vi "Main.vi"(8 "error in (no error)":errorcluster, 11 "AOTFBase in":refnum<class "AOTF.lvclass">) -> (0 "error out":errorcluster, 3 "component":refnum<class "AOTF.lvclass">)   [LabVIEW 2012, in "AOTF.lvclass"]
doc: "Main VI of the component."
uses:
  AOTF.lvclass
  Controls/laser line enum.ctl
  <vilib>/Distrio/Murmex/Murmex/command_enum.ctl
  AOTF.lvclass/AOTF.ctl
  <vilib>/Distrio/Murmex/InitialiseMessage/InitialiseMessage.lvclass
  <vilib>/Distrio/Murmex/ConfigureMessage/ConfigureMessage.lvclass
  <vilib>/Distrio/Murmex/TerminateMessage/TerminateMessage.lvclass
  <vilib>/Distrio/Murmex/Murmex/update_cluster.ctl
  <vilib>/Distrio/Murmex/GenericMessage/GenericMessage.lvclass
  <vilib>/Distrio/Murmex/Murmex/Set configure at initialise.vi
  <vilib>/Distrio/Murmex/Murmex/Set log reference.vi
  <vilib>/Distrio/Murmex/Murmex/Set VI reference.vi
  <vilib>/Distrio/Murmex/Murmex/Get ID.vi
  <vilib>/Distrio/Murmex/Message/Add or replace parameter.vi
  <vilib>/Distrio/Murmex/Murmex/Murmex.lvclass
  <vilib>/Distrio/Murmex/Message/Message.lvclass
panel:
  in  "button::configure":bool
  in  "button::quit":bool
  out "terminate?":bool=TRUE
  in  "Tab Control":enum32{"Main", "Debug"}(tab)
  in  "PowerPercentage":dbl(knob)=50.0 min=0.0 max=100.0 step=5.0 scale=0.0..100.0
  in  "button::status":bool
  in  "Line On/Off":bool
  in  "button::shutter":bool
  in  "Frequency":T1=103.5 items=["405nm"=150.3, "445nm"=128.71, "491nm"=110.257, "515nm"=103.5, "561nm"=93.2]
  in  "Line number":u32=1 min=1 max=8 step=1
  out "Last read buffer":string="l1F103.500P12.8S1\n\r"
  out "log":string="\r\n11:11:41.970 05/12/2013: initialise from AOTF to AOTF\r\n11:11:42.586 05/12/2013: inform from AOTF to AOTF\r\n11:11:43.913 05/12/2013: update from AOTF to AOTF\r\n11:11:45.142 05/12/2013: generic (shutter_off) from AOTF to AOTF\r\n11:11:45.270 05/12/2013: generic (shutter_on) from AOTF to AOTF\r\n11:11:45.902 05/12/2013: generic (shutter_off) from AOTF to AOTF\r\n11:11:45.932 05/12/2013: inspect from AOTF to AOTF\r\n11:11:48.013 05/12/2013: configure from AOTF to AOTF\r\n11:11:52.003 05/12/2013: inform from AOTF to AOTF\r\n11:11:58.521 05/12/2013: initialise from AOTF to AOTF\r\n11:11:58.561 05/12/2013: inform from AOTF to AOTF\r\n11:11:58.695 05/12/2013: inform from AOTF to AOTF\r\n11:12:02.089 05/12/2013: update from AOTF to AOTF\r\n11:12:02.308 05/12/2013: inspect from AOTF to AOTF\r\n11:12:02.364 05/12/2013: inform from AOTF to AOTF\r\n11:12:05.062 05/12/2013: generic (shutter_on) from AOTF to AOTF\r\n11:12:06.690 05/12/2013: update from AOTF to AOTF\r\n11:12:06.909 05/12/2013: inspect from AOTF to AOTF\r\n11:12:06.964 05/12/2013: inform from AOTF to AOTF\r\n11:12:07.770 05/12/2013: update from AOTF to AOTF\r\n11:12:07.989 05/12/2013: inspect from AOTF to AOTF\r\n11:12:08.044 05/12/2013: inform from AOTF to AOTF\r\n11:12:08.627 05/12/2013: update from AOTF to AOTF\r\n11:12:08.846 05/12/2013: inspect from AOTF to AOTF\r\n11:12:08.900 05/12/2013: inform from AOTF to AOTF\r\n11:12:09.290 05/12/2013: update from AOTF to AOTF\r\n11:12:09.508 05/12/2013: inspect from AOTF to AOTF\r\n11:12:09.563 05/12/2013: inform from AOTF to AOTF\r\n11:12:10.154 05/12/2013: update from AOTF to AOTF\r\n11:12:10.373 05/12/2013: inspect from AOTF to AOTF\r\n11:12:10.430 05/12/2013: inform from AOTF to AOTF\r\n11:12:20.953 05/12/2013: update from AOTF to AOTF\r\n11:12:21.172 05/12/2013: inspect from AOTF to AOTF\r\n11:12:21.227 05/12/2013: inform from AOTF to AOTF\r\n11:12:22.057 05/12/2013: update from AOTF to AOTF\r\n11:12:22.276 05/12/2013: inspect from AOTF to AOTF\r\n11:12:22.330 05/12/2013: inform from AOTF to AOTF\r\n11:12:22.841 05/12/2013: update from AOTF to AOTF\r\n11:12:23.060 05/12/2013: inspect from AOTF to AOTF\r\n11:12:23.114 05/12/2013: inform from AOTF to AOTF\r\n11:12:23.449 05/12/2013: update from AOTF to AOTF\r\n11:12:23.668 05/12/2013: inspect from AOTF to AOTF\r\n11:12:23.724 05/12/2013: inform from AOTF to AOTF\r\n11:12:24.514 05/12/2013: update from AOTF to AOTF\r\n11:12:24.733 05/12/2013: inspect from AOTF to AOTF\r\n11:12:24.789 05/12/2013: inform from AOTF to AOTF\r\n11:12:25.098 05/12/2013: update from AOTF to AOTF\r\n11:12:25.317 05/12/2013: inspect from AOTF to AOTF\r\n11:12:25.371 05/12/2013: inform from AOTF to AOTF\r\n11:12:26.482 05/12/2013: update from AOTF to AOTF\r\n11:12:26.701 05/12/2013: inspect from AOTF to AOTF\r\n11:12:26.755 05/12/2013: inform from AOTF to AOTF\r\n11:12:27.154 05/12/2013: update from AOTF to AOTF\r\n11:12:27.373 05/12/2013: inspect from AOTF to AOTF\r\n11:12:27.428 05/12/2013: inform from AOTF to AOTF\r\n11:12:27.666 05/12/2013: update from AOTF to AOTF\r\n11:12:27.885 05/12/2013: inspect from AOTF to AOTF\r\n11:12:27.944 05/12/2013: inform from AOTF to AOTF\r\n11:12:33.380 05/12/2013: update from AOTF to AOTF\r\n11:12:33.484 05/12/2013: update from AOTF to AOTF\r\n11:12:33.603 05/12/2013: inspect from AOTF to AOTF\r\n11:12:33.611 05/12/2013: update from AOTF to AOTF\r\n11:12:33.684 05/12/2013: update from AOTF to AOTF\r\n11:12:33.740 05/12/2013: update from AOTF to AOTF\r\n11:12:33.827 05/12/2013: inspect from AOTF to AOTF\r\n11:12:33.835 05/12/2013: update from AOTF to AOTF\r\n11:12:33.897 05/12/2013: inform from AOTF to AOTF\r\n11:12:33.903 05/12/2013: update from AOTF to AOTF\r\n11:12:33.940 05/12/2013: update from AOTF to AOTF\r\n11:12:34.085 05/12/2013: update from AOTF to AOTF\r\n11:12:34.119 05/12/2013: inspect from AOTF to AOTF\r\n11:12:34.292 05/12/2013: update from AOTF to AOTF\r\n11:12:34.336 05/12/2013: inspect from AOTF to AOTF\r\n11:12:34.553 05/12/2013: inspect from AOTF to AOTF\r\n11:12:34.608 05/12/2013: inform from AOTF to AOTF\r\n11:12:34.739 05/12/2013: update from AOTF to AOTF\r\n11:12:34.771 05/12/2013: update from AOTF to AOTF\r\n11:12:34.826 05/12/2013: inspect from AOTF to AOTF\r\n11:12:34.834 05/12/2013: update from AOTF to AOTF\r\n11:12:34.867 05/12/2013: update from AOTF to AOTF\r\n11:12:34.931 05/12/2013: update from AOTF to AOTF\r\n11:12:34.979 05/12/2013: update from AOTF to AOTF\r\n11:12:35.003 05/12/2013: update from AOTF to AOTF\r\n11:12:35.027 05/12/2013: update from AOTF to AOTF\r\n11:12:35.041 05/12/2013: update from AOTF to AOTF\r\n11:12:35.051 05/12/2013: inspect from AOTF to AOTF\r\n11:12:35.066 05/12/2013: update from AOTF to AOTF\r\n11:12:35.116 05/12/2013: update from AOTF to AOTF\r\n11:12:35.171 05/12/2013: update from AOTF to AOTF\r\n11:12:35.211 05/12/2013: update from AOTF to AOTF\r\n11:12:35.273 05/12/2013: inspect from AOTF to AOTF\r\n11:12:35.287 05/12/2013: update from AOTF to AOTF\r\n11:12:35.475 05/12/2013: update from AOTF to AOTF\r\n11:12:35.495 05/12/2013: inspect from AOTF to AOTF\r\n11:12:35.549 05/12/2013: inform from AOTF to AOTF\r\n11:12:35.764 05/12/2013: inspect from AOTF to AOTF\r\n11:12:35.819 05/12/2013: inform from AOTF to AOTF\r\n11:12:35.861 05/12/2013: update from AOTF to AOTF\r\n11:12:35.877 05/12/2013: inform from AOTF to AOTF\r\n11:12:35.947 05/12/2013: update from AOTF to AOTF\r\n11:12:36.067 05/12/2013: update from AOTF to AOTF\r\n11:12:36.100 05/12/2013: inspect from AOTF to AOTF\r\n11:12:36.235 05/12/2013: update from AOTF to AOTF\r\n11:12:36.317 05/12/2013: inspect from AOTF to AOTF\r\n11:12:36.371 05/12/2013: inform from AOTF to AOTF\r\n11:12:36.587 05/12/2013: inspect from AOTF to AOTF\r\n11:12:36.771 05/12/2013: update from AOTF to AOTF\r\n11:12:36.804 05/12/2013: inspect from AOTF to AOTF\r\n11:12:37.020 05/12/2013: inspect from AOTF to AOTF\r\n11:12:37.238 05/12/2013: inspect from AOTF to AOTF\r\n11:12:37.456 05/12/2013: inspect from AOTF to AOTF\r\n11:12:37.673 05/12/2013: inspect from AOTF to AOTF\r\n11:12:37.891 05/12/2013: inspect from AOTF to AOTF\r\n11:12:37.946 05/12/2013: inform from AOTF to AOTF\r\n11:12:38.161 05/12/2013: inspect from AOTF to AOTF\r\n11:12:38.379 05/12/2013: inspect from AOTF to AOTF\r\n11:12:38.597 05/12/2013: inspect from AOTF to AOTF\r\n11:12:38.815 05/12/2013: inspect from AOTF to AOTF\r\n11:12:38.871 05/12/2013: inform from AOTF to AOTF\r\n11:12:39.086 05/12/2013: inspect from AOTF to AOTF\r\n11:12:39.303 05/12/2013: inspect from AOTF to AOTF\r\n11:12:39.363 05/12/2013: inform from AOTF to AOTF\r\n11:12:39.417 05/12/2013: inform from AOTF to AOTF\r\n11:12:39.633 05/12/2013: inspect from AOTF to AOTF\r\n11:12:39.852 05/12/2013: inspect from AOTF to AOTF\r\n11:12:40.069 05/12/2013: inspect from AOTF to AOTF\r\n11:12:40.124 05/12/2013: inform from AOTF to AOTF\r\n11:12:40.339 05/12/2013: inspect from AOTF to AOTF\r\n11:12:40.395 05/12/2013: inform from AOTF to AOTF\r\n11:12:40.448 05/12/2013: inform from AOTF to AOTF\r\n11:12:40.663 05/12/2013: inspect from AOTF to AOTF\r\n11:12:40.718 05/12/2013: inform from AOTF to AOTF\r\n11:12:40.770 05/12/2013: inform from AOTF to AOTF\r\n11:12:40.824 05/12/2013: inform from AOTF to AOTF\r\n11:12:40.877 05/12/2013: inform from AOTF to AOTF\r\n11:12:40.930 05/12/2013: inform from AOTF to AOTF\r\n11:12:40.982 05/12/2013: inform from AOTF to AOTF\r\n11:12:41.034 05/12/2013: inform from AOTF to AOTF\r\n11:12:41.092 05/12/2013: inform from AOTF to AOTF\r\n11:12:41.144 05/12/2013: inform from AOTF to AOTF\r\n11:12:41.196 05/12/2013: inform from AOTF to AOTF\r\n11:12:41.249 05/12/2013: inform from AOTF to AOTF\r\n11:12:41.307 05/12/2013: inform from AOTF to AOTF\r\n11:12:41.366 05/12/2013: inform from AOTF to AOTF\r\n11:12:41.424 05/12/2013: inform from AOTF to AOTF\r\n11:12:41.478 05/12/2013: inform from AOTF to AOTF\r\n11:12:41.533 05/12/2013: inform from AOTF to AOTF\r\n11:12:41.589 05/12/2013: inform from AOTF to AOTF\r\n11:12:42.246 05/12/2013: terminate from AOTF to AOTF"
  in  "component ID":string="AOTF"
  in  "button::send":bool
  in  "command":T2
  in  "Generic command":string
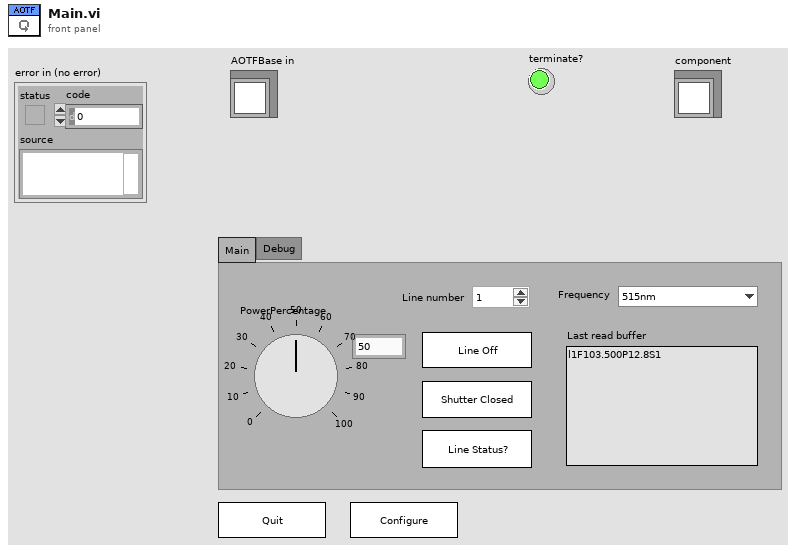
[diagram p1: front panel]
types:
  T1 = typedef "AOTF.lvclass/laser line enum.ctl" = dbl
  T2 = typedef "Murmex.lvlib/Murmex.lvclass/command_enum.ctl" = enum16{"null", "initialise", "reset", "terminate", "acknowledge", "update", "inspect", "inform", "proceed", "start", "stop", "fetch", "configure", "generic"}
  T3 = enum8{"Enabled", "Disabled", "Disabled and Grayed Out"}
  T4 = typedef "Murmex.lvlib/Murmex.lvclass/update_cluster.ctl" = cluster{"target ID":string, "key chains":string[], "values":variant[]}
  T5 = typedef "Murmex.lvclass/command_enum.ctl" = enum16{"null", "initialise", "reset", "terminate", "acknowledge", "update", "inspect", "inform", "proceed", "start", "stop", "fetch", "configure", "generic"}
  T6 = typedef "Murmex.lvclass/Event type enumerations.ctl" = enum16{"before", "after"}
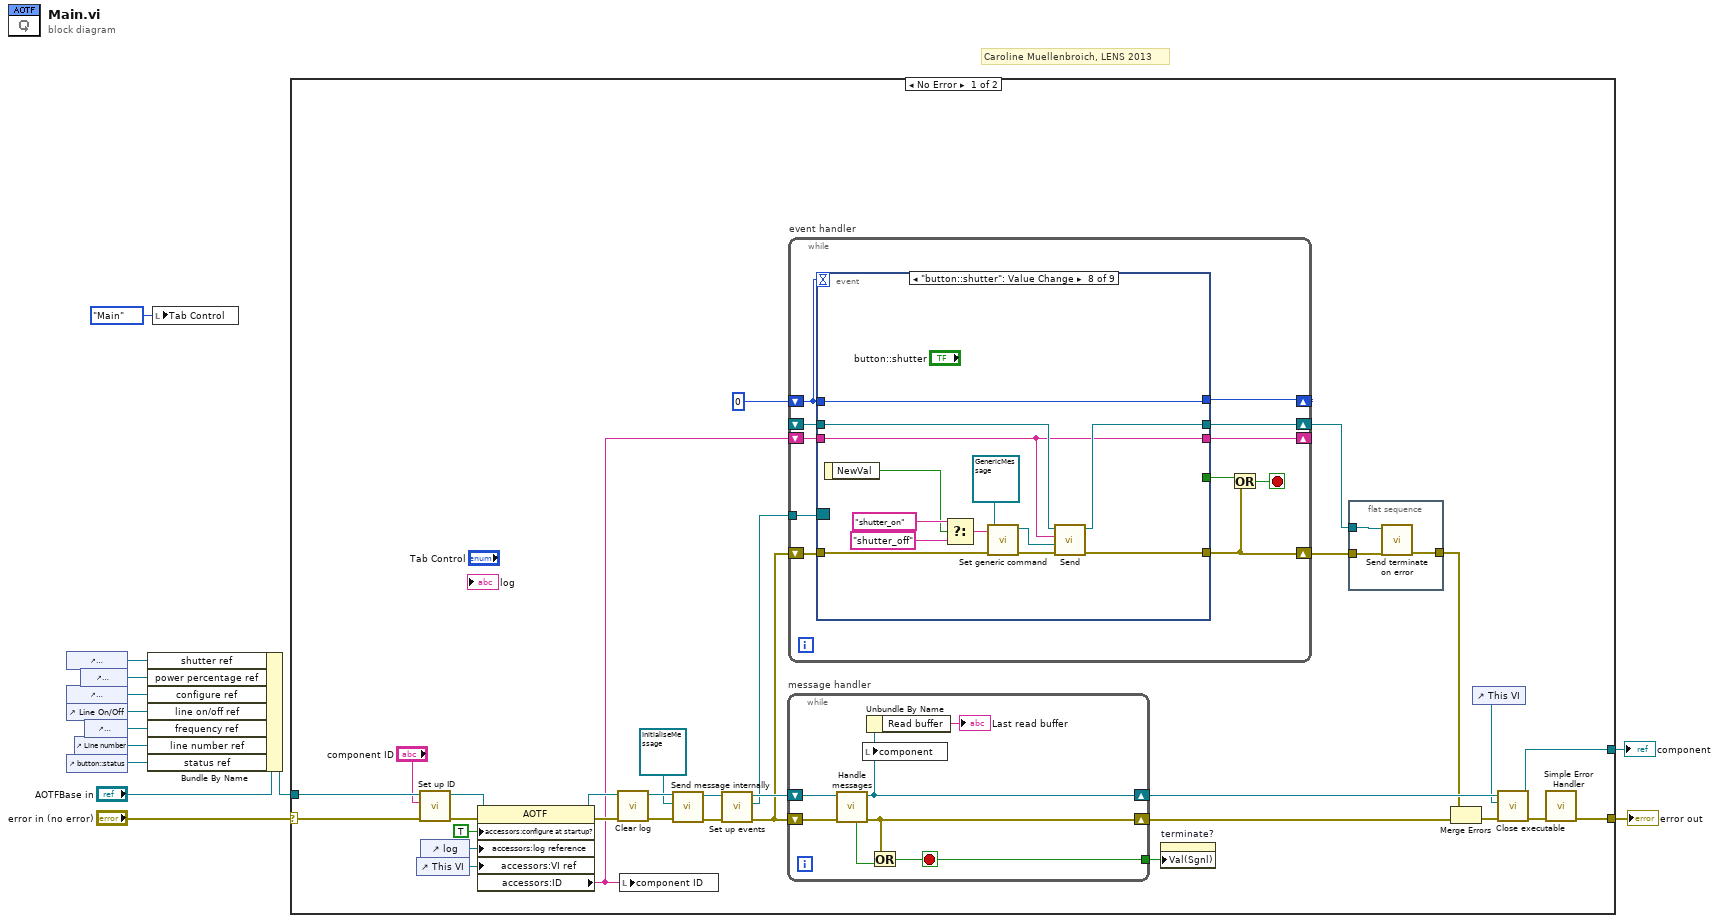
[diagram p0: block diagram]
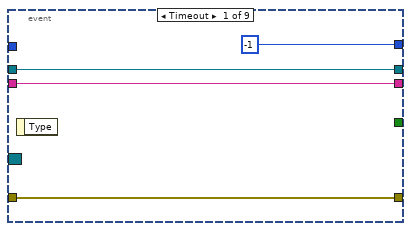
[diagram p2: hidden frame]
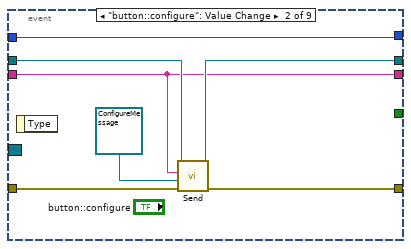
[diagram p3: hidden frame]
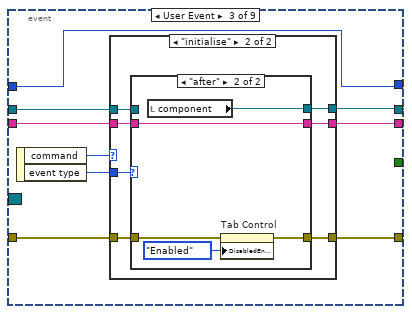
[diagram p4: hidden frame]
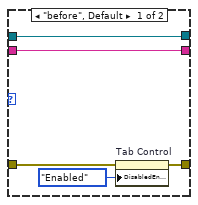
[diagram p6: hidden frame]
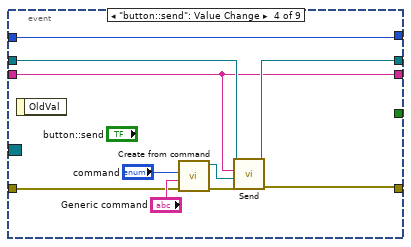
[diagram p7: hidden frame]
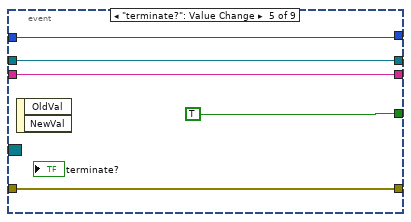
[diagram p8: hidden frame]
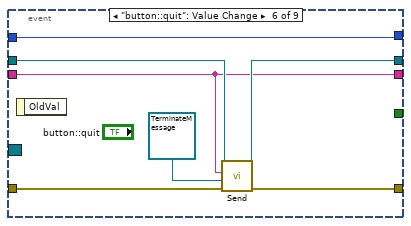
[diagram p9: hidden frame]
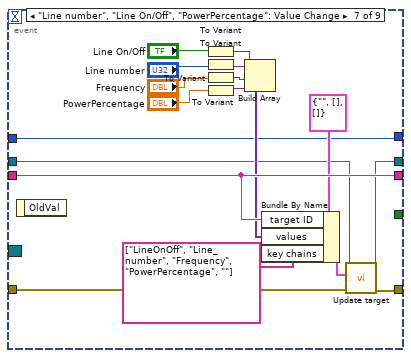
[diagram p10: hidden frame]
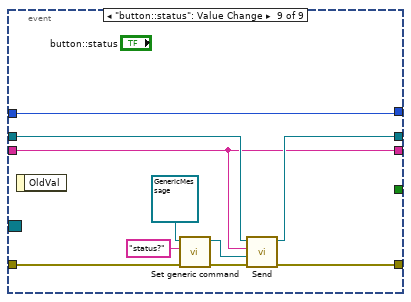
[diagram p11: hidden frame]
diagram:
  # "Caroline Muellenbroich, LENS 2013"
  n1 = control-ref of="button::shutter"() -> (w4:refnum<vi>)
  n2 = control-ref of="button::configure"() -> (w7:refnum<vi>)
  n3 = control-ref of="Line On/Off"() -> (w2:refnum<vi>)
  n4 = control-ref of="button::status"() -> (w1:refnum<vi>)
  n5 = control-ref of="Line number"() -> (w5:refnum<vi>)
  n6 = control-ref of="PowerPercentage"() -> (w3:refnum<vi>)
  n7 = control-ref of="Frequency"() -> (w6:refnum<vi>)
  n8 = Bundle By Name(cluster="AOTFBase in", "shutter ref"=w4, "power percentage ref"=w3, "configure ref"=w7, "line on/off ref"=w2, "frequency ref"=w6, "line number ref"=w5, "status ref"=w1) -> (w8:refnum<class "AOTF.lvclass">)
  n9 = local write "Tab Control"(enum32{"Main", "Debug"}."Main" ("Tab Control")) -> ()
  n10 = case shown="No Error" "error in (no error)" {
    selector: "error in (no error)" -> [w17 w170]
    tunnel: w8 -> [w44 w169]
    tunnel: [w27 w169] -> w13
    tunnel: [w23 w170] -> w12
    frame No Error {
      n11 = control-ref of="This VI"() -> (w39:refnum<vi>)
      n12 = call <vilib>:"Set up ID.vi"("error in (no error)"=w17, "component ID"="component ID", "MurmexBase in"=w44) -> ("error out"=w43:errorcluster, "MurmexBase out"=w42:refnum<class "AOTF.lvclass">)  [unwired: 6 in, 1 out]
      n13 = control-ref of="log"() -> (w40:refnum<vi>)
      n14 = property class="AOTF"(reference=w42, error in=w43, "accessors:configure at startup?"=TRUE ("configure at startup?"), "accessors:log reference"=w40, "accessors:VI ref"=w39) -> (reference out=w36:refnum<class "AOTF.lvclass">, error out=w38:errorcluster, "accessors:ID"=w16:string)
      n15 = call <vilib>:"Clear log.vi"("error in (no error)"=w38, "MurmexBase in"=w36) -> ("error out"=w37:errorcluster, "MurmexBase out"=w35:refnum<class "AOTF.lvclass">)  [unwired: 8 in]
      n16 = local write "component ID"(w16) -> ()
      n17 = call <vilib>:"Send message internally.vi"("error in (no error)"=w37, "Message"=refnum<class "InitialiseMessage.lvclass"> refnum ("Murmex.lvlib:InitialiseMessage"), "Murmex in"=w35) -> ("error out"=w34:errorcluster, "Murmex out"=w33:refnum<class "AOTF.lvclass">)  [unwired: 7 in]
      n18 = call <vilib>:"Set up events.vi"("error in (no error)"=w34, "MurmexBase in"=w33) -> ("error out"=w26:errorcluster, "Event Registration Refnum"=w25:refnum<event-registration>, "MurmexBase out"=w32:refnum<class "AOTF.lvclass">)  [unwired: 7 in]
      n19 = while "message handler" {
        shift-right: [w163] -> w28
        shift-left: w32 -> [w167]
        shift-right: [w166] -> w29
        shift-left: w26 -> [w168]
        tunnel: [w164] -> w24
        stop <- w164 stop-if-true
        n20 = call <vilib>:"Handle messages.vi"("error in (no error)"=w168, "Murmex in"=w167) -> ("error out"=w166:errorcluster, "Murmex out"=w163:refnum<class "AOTF.lvclass">, "terminated?"=w165:bool)  [unwired: 7 in]
        n21 = local write "component"(w163) -> ()
        n22 = Unbundle By Name(w163) -> ("Read buffer"=→"Last read buffer":string)
        n23 = Or(x=w166, y=w165) -> (x .or. y?=w164:bool)
      }
      n24 = while "event handler" {
        tunnel: w25 -> [w58]
        shift-right: [w51] -> w21
        shift-left: w26 -> [w57]
        shift-right: [w53] -> _
        shift-left: w16 -> [w56]
        shift-right: [w55] -> w19
        shift-left: _ -> [w54]
        shift-right: [w49] -> _
        shift-left: 0 -> [w48]
        stop <- w52 stop-if-true
        n25 = event shown="[7] \"button::shutter\": Value Change" {
          selector: w58 -> [_ _ _ _ _ _ _ _ _]
          dyn-events: _ -> [_ _ _ _ _ _ _ _ _]
          timeout: w48 -> [_ _ _ _ _ _ _ _ _]
          tunnel: w57 -> [w60 w69 w76 w105 w113 w120 w137 w149 w159]
          tunnel: [w60 w68 w75 w104 w113 w119 w138 w150 w160] -> w51
          tunnel: w56 -> [w62 w64 w74 w100 w111 w115 w136 w142 w154]
          tunnel: [w61 w66 w73 w102 w110 w117 w130 w146 w156] -> w55
          tunnel: w54 -> [w61 w67 w72 w103 w110 w118 w131 w147 w157]
          tunnel: [w62 w64 w71 w100 w111 w115 w136 w142 w154] -> w53
          tunnel: [_ _ _ _ TRUE _ _ _ _] -> w50
          tunnel: w48 -> [_ w65 w70 w101 w109 w116 w123 w140 w153]
          tunnel: [-1 w65 w70 w101 w109 w116 w123 w140 w153] -> w49
          event Timeout {
            n26 = event-data() -> ()  [unwired: 1 in, 1 out]
          }
          event "button::configure": Value Change {
            n27 = event-data() -> ()  [unwired: 1 in, 1 out]
            n28 = call <vilib>:"Send.vi"("error in (no error)"=w69, "Message"=refnum<class "ConfigureMessage.lvclass"> refnum ("Murmex.lvlib:ConfigureMessage"), "recipient"=w64, "Murmex in"=w67) -> ("error out"=w68:errorcluster, "Murmex out"=w66:refnum<class "Murmex.lvclass">)  [unwired: 6 in]
          }
          event User Event {
            n29 = event-data() -> ("command"=w78:T5, "event type"=w77:T6)  [unwired: 1 in]
            n30 = case shown="\"initialise\"" w78 {
              tunnel: w77 -> [_ w88]
              tunnel: w76 -> [w79 w87]
              tunnel: [w79 w86] -> w75
              tunnel: w74 -> [w81 w85]
              tunnel: [w80 w84] -> w73
              tunnel: w72 -> [w80 w83]
              tunnel: [w81 w82] -> w71
              frame "null", Default {
              }
              frame "initialise" {
                n31 = case shown="\"after\"" w88 {
                  tunnel: [w92 w97] -> w86
                  tunnel: w87 -> [w93 w98]
                  tunnel: w85 -> [w90 w94]
                  tunnel: [w89 w96] -> w84
                  tunnel: w83 -> [w89 _]
                  tunnel: [w90 w94] -> w82
                  frame "before", Default {
                    n32 = property on="Tab Control" class="TabCtl (strict)"(error in=w93, "DisabledEnum"=T3."Enabled" ("Disabled")) -> (error out=w92:errorcluster)  [unwired: 1 in, 1 out]
                  }
                  frame "after" {
                    n33 = local read "component"() -> (w96:refnum<class "AOTF.lvclass">)
                    n34 = property on="Tab Control" class="TabCtl (strict)"(error in=w98, "DisabledEnum"=T3."Enabled" ("Disabled")) -> (error out=w97:errorcluster)  [unwired: 1 in, 1 out]
                  }
                }
              }
            }
          }
          event "button::send": Value Change {
            n35 = event-data() -> ()  [unwired: 1 in, 1 out]
            n36 = call <vilib>:"Create from command.vi"("error in (no error)"=w105, "generic command"="Generic command", "command"="command") -> ("error out"=w107:errorcluster, "Message out"=w106:refnum<class "Message.lvclass">)  [unwired: 7 in]
            n37 = call <vilib>:"Send.vi"("error in (no error)"=w107, "Message"=w106, "recipient"=w100, "Murmex in"=w103) -> ("error out"=w104:errorcluster, "Murmex out"=w102:refnum<class "Murmex.lvclass">)  [unwired: 6 in]
          }
          event "terminate?": Value Change {
            n38 = event-data() -> ()  [unwired: 1 in, 2 out]
          }
          event "button::quit": Value Change {
            n39 = event-data() -> ()  [unwired: 1 in, 1 out]
            n40 = call <vilib>:"Send.vi"("error in (no error)"=w120, "Message"=refnum<class "TerminateMessage.lvclass"> refnum ("Murmex.lvlib:TerminateMessage"), "recipient"=w115, "Murmex in"=w118) -> ("error out"=w119:errorcluster, "Murmex out"=w117:refnum<class "Murmex.lvclass">)  [unwired: 6 in]
          }
          event "Line number", "Line On/Off", "PowerPercentage": Value Change {
            n41 = event-data() -> ()  [unwired: 1 in, 1 out]
            n42 = To Variant(anything="Line On/Off") -> (Variant=w129:variant)
            n43 = To Variant(anything="Line number") -> (Variant=w126:variant)
            n44 = To Variant(anything="Frequency") -> (Variant=w127:variant)
            n45 = To Variant(anything="PowerPercentage") -> (Variant=w128:variant)
            n46 = Build Array(w129, w126, w127, w128) -> (w132:variant[])
            n47 = Bundle By Name(cluster=T4 {"target ID"="", "key chains"=[], "values"=[]} ("update cluster"), "target ID"=w136, "values"=w132, "key chains"=string[] ["LineOnOff", "Line_number", "Frequency", "PowerPercentage", ""]) -> (w135:T4)
            n48 = call <vilib>:"Update target.vi"("error in (no error)"=w137, "update cluster"=w135, "MurmexBase in"=w131) -> ("error out"=w138:errorcluster, "MurmexBase out"=w130:refnum<class "Murmex.lvclass">)  [unwired: 7 in]
          }
          event "button::shutter": Value Change {
            n49 = event-data() -> ("NewVal"=w141:bool)  [unwired: 1 in]
            n50 = Select(t="shutter_on" ("generic command"), s=w141, f="shutter_off" ("generic command")) -> (s? t:f=w143:string)
            n51 = call <vilib>:"Set generic command.vi"("error in (no error)"=w149, "generic command"=w143, "GenericMessage in"=refnum<class "GenericMessage.lvclass"> refnum ("Murmex.lvlib:GenericMessage")) -> ("error out"=w148:errorcluster, "GenericMessage out"=w151:refnum<class "GenericMessage.lvclass">)  [unwired: 7 in]
            n52 = call <vilib>:"Send.vi"("error in (no error)"=w148, "Message"=w151, "recipient"=w142, "Murmex in"=w147) -> ("error out"=w150:errorcluster, "Murmex out"=w146:refnum<class "Murmex.lvclass">)  [unwired: 6 in]
          }
          event "button::status": Value Change {
            n53 = event-data() -> ()  [unwired: 1 in, 1 out]
            n54 = call <vilib>:"Set generic command.vi"("error in (no error)"=w159, "generic command"="status?", "GenericMessage in"=refnum<class "GenericMessage.lvclass"> refnum ("Murmex.lvlib:GenericMessage")) -> ("error out"=w158:errorcluster, "GenericMessage out"=w161:refnum<class "GenericMessage.lvclass">)  [unwired: 7 in]
            n55 = call <vilib>:"Send.vi"("error in (no error)"=w158, "Message"=w161, "recipient"=w154, "Murmex in"=w157) -> ("error out"=w160:errorcluster, "Murmex out"=w156:refnum<class "Murmex.lvclass">)  [unwired: 6 in]
          }
        }
        n56 = Or(x=w50, y=w51) -> (x .or. y?=w52:bool)
      }
      n57 = property on="terminate?" class="Bool (strict)"("Val(Sgnl)"=w24) -> ()  [unwired: 2 in, 2 out]
      n58 = flat-sequence {
        tunnel: w21 -> [w46]
        tunnel: [w47] -> w20
        tunnel: w19 -> [w45]
        frame #0 {
          n59 = call <vilib>:"Send terminate on error.vi"("error in (no error)"=w46, "Murmex in"=w45) -> ("error out"=w47:errorcluster)  [unwired: 8 in, 1 out]
        }
      }
      n60 = Merge Errors(w20, w29) -> (w30:errorcluster)
      n61 = control-ref of="This VI"() -> (w18:refnum<vi>)
      n62 = call <vilib>:"Close executable.vi"("error in (no error)"=w30, "main VI ref (optional)"=w18, "MurmexBase in"=w28) -> ("error out"=w31:errorcluster, "MurmexBase out"=w27:refnum<class "AOTF.lvclass">)  [unwired: 7 in]
      n63 = call <vilib>:"Simple Error Handler.vi"("error in (no error)"=w31) -> ("error out"=w23:errorcluster)  [unwired: 4 in, 4 out]
    }
    frame Error {
    }
  }
  "error out" <- w12
  "component" <- w13
